vi "Set Data Server Options.vi"(6 "launch data viewer":bool, 8 "error in":errorcluster, 9 "data server frequency (Hz)":dbl, 10 "enable data server":bool, 11 "data sharing framework custom device in":T1 format="%.0x") -> (0 "error out":errorcluster, 3 "data sharing framework custom device out":T1 format="%.0x")   [LabVIEW 2017, in "Data Sharing Framework Custom Device Scripting.lvlib"]
uses:
  Data Sharing Framework Custom Device Scripting.lvlib
  <vilib>/NI Veristand/Custom Device API/Custom Device Item Ref.ctl
  Shared/DSF Shared.lvlib
  <vilib>/NI Veristand/Custom Device API/Custom Device API.lvlib
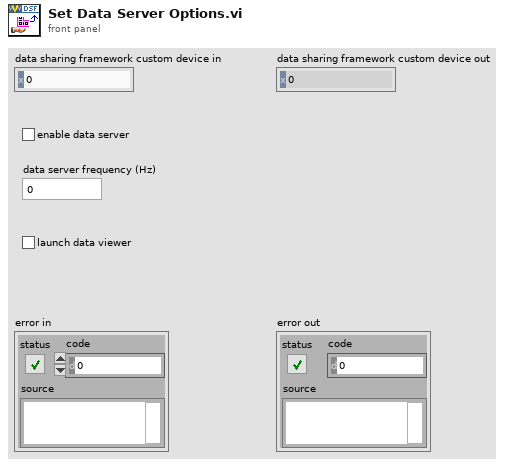
[diagram p1: front panel]
types:
  T1 = typedef "Custom Device API.lvlib/Custom Device Item Ref.ctl" = u64
  T2 = typedef "DSF Core.lvlibp/Framework.lvclass/Framework Options.ctl" = cluster{"FIFO Options":T3, "Thread Options":T4, "Plugin Options":T5, "Performance Options":T6, "Data Server Options":T7}
  T3 = typedef "DSF Core.lvlibp/Framework.lvclass/DSF FIFO Options.ctl" = cluster{"Infinite Timeouts":bool}
  T4 = typedef "DSF Core.lvlibp/Thread.lvclass/Thread Options.ctl" = cluster{"Show FP On Call":bool, "Close FP After Call":bool, "Allow Debugging":bool}
  T5 = typedef "DSF Core.lvlibp/Framework.lvclass/DSF Plugin Options.ctl" = cluster{"Default Components":bool}
  T6 = typedef "DSF Core.lvlibp/DSF Performance Options.ctl" = cluster{"Measure Period":bool, "Measure Rx/Tx Duration":bool}
  T7 = typedef "DSF Core.lvlibp/Framework.lvclass/Data Server Options.ctl" = cluster{"Enable Data Server":bool, "Period":u32}
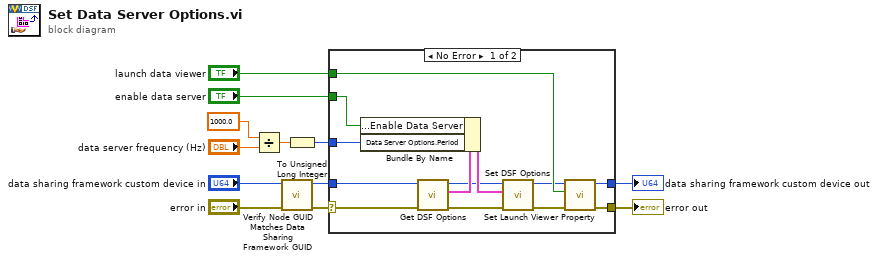
[diagram p0: block diagram]
diagram:
  n1 = Divide(x=1000.0 ("y"), y="data server frequency (Hz)") -> (x/y=w11:dbl)
  n2 = call "Verify Node GUID Matches Data Sharing Framework GUID.vi"("error in"="error in", "data sharing framework custom device in"="data sharing framework custom device in") -> ("error out"=w2:errorcluster, "data sharing framework custom device out"=w1:T1)  [unwired: 8 in]
  n3 = To Unsigned Long Integer(number=w11) -> (unsigned 32bit integer=w10:u32)
  n4 = case shown="No Error" w2 {
    selector: w2 -> [w14 w26]
    tunnel: w10 -> [w24 _]
    tunnel: "enable data server" -> [w20 _]
    tunnel: "launch data viewer" -> [w19 _]
    tunnel: [w16 w27] -> w6
    tunnel: [w15 w26] -> w5
    tunnel: w1 -> [w13 w27]
    frame No Error {
      n5 = call "Get DSF Options.vi"("error in (no error)"=w14, "Item Ref in"=w13) -> ("error out"=w25:errorcluster, "options"=w23:T2, "Item Ref out"=w21:T1)  [unwired: 7 in]
      n6 = Bundle By Name(cluster=w23, "Data Server Options.Enable Data Server"=w20, "Data Server Options.Period"=w24) -> (w22:T2)
      n7 = call "Set DSF Options.vi"("error in (no error)"=w25, "options"=w22, "Item Ref in"=w21) -> ("error out"=w17:errorcluster, "Item Ref out"=w18:T1)  [unwired: 7 in]
      n8 = call "Set Launch Viewer Property.vi"("error in (no error)"=w17, "launch viewer"=w19, "Item Ref in"=w18) -> ("error out"=w15:errorcluster, "Item Ref out"=w16:T1)  [unwired: 7 in]
    }
    frame Error {
    }
  }
  "data sharing framework custom device out" <- w6
  "error out" <- w5
